vi "2 Sync - Digital Trigger.vi"() -> ()   [LabVIEW 2023]
doc: "This example demonstrates how to acquire a single buffer of voltage measurements using a DAQmx device.\n\nFor instructions on how to connect your signals to the DAQ device, refer to your device documentation."
uses:
  <vilib>/DAQmx/create/channels.llb/DAQmx Create Channel (AI-Voltage-Basic).vi
  <vilib>/DAQmx/configure/timing.llb/DAQmx Timing (Sample Clock).vi
  <vilib>/DAQmx/read.llb/DAQmx Read (Analog Wfm 1Chan NSamp).vi
  <vilib>/Analysis/NI_AALBase.lvlib
  <resource>/objmgr/daqmx.rc
  <vilib>/DAQmx/configure/trigger.llb/DAQmx Start Trigger (Digital Edge).vi
  <vilib>/DAQmx/write.llb/DAQmx Write (Digital Bool 1Line 1Point).vi
  <vilib>/DAQmx/configure/timing.llb/DAQmx Timing (Implicit).vi
  <vilib>/DAQmx/create/channels.llb/DAQmx Create Channel (CO-Pulse Generation-Frequency).vi
  <vilib>/DAQmx/create/channels.llb/DAQmx Create Channel (DO-Digital Output).vi
panel:
  in  "Trigger Output: Line":tag="MIODAQ/port0/line2"
  in  "Device 2: Trigger Input":tag="/cDAQ9189-2628AACMod5/PFI4"
  in  "Device 1: Trigger Input":tag="/MIODAQ/PFI4"
  in  "Square Wave Output: Terminal":tag="/MIODAQ/PFI0"
  in  "Square Wave Output: Source":tag="MIODAQ/ctr0"
  out "Progress":i32(slide) scale=0.0..9.0
  out "Standard Deviation":dbl format="%0.2f"
  out "Range":dbl
  out "Mean":dbl format="%0.2f"
  out "Skew":dbl
  in  "Device 2: Analog Input Channel":tag="cDAQ9189-2628AACMod1/ai0"
  out "Waveform Graph":waveform(dbl)[](graph)
  in  "Device 1: Analog Input Channel":tag="MIODAQ/ai0"
  # "Channel Settings"
  # "Acquired Data"
  # "Trigger Acq Settings"
  # "Output Signal Settings"
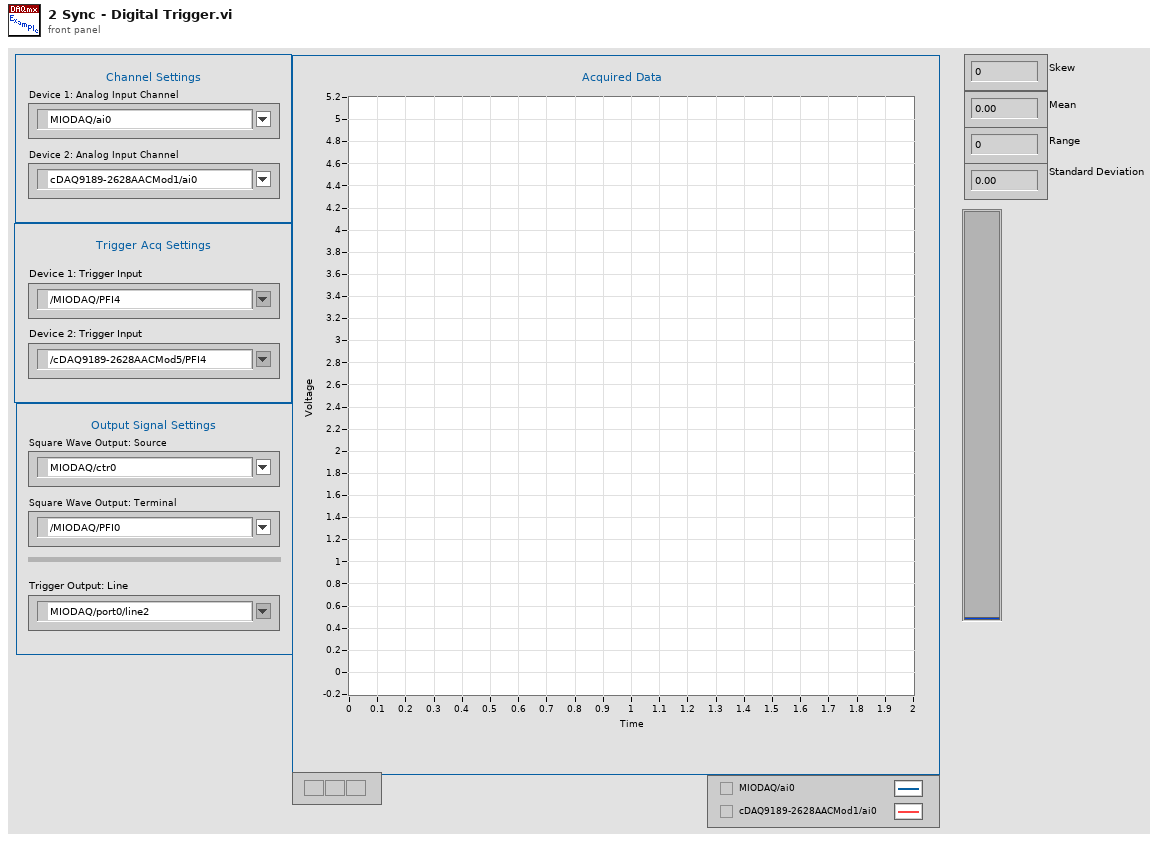
[diagram p1: front panel]
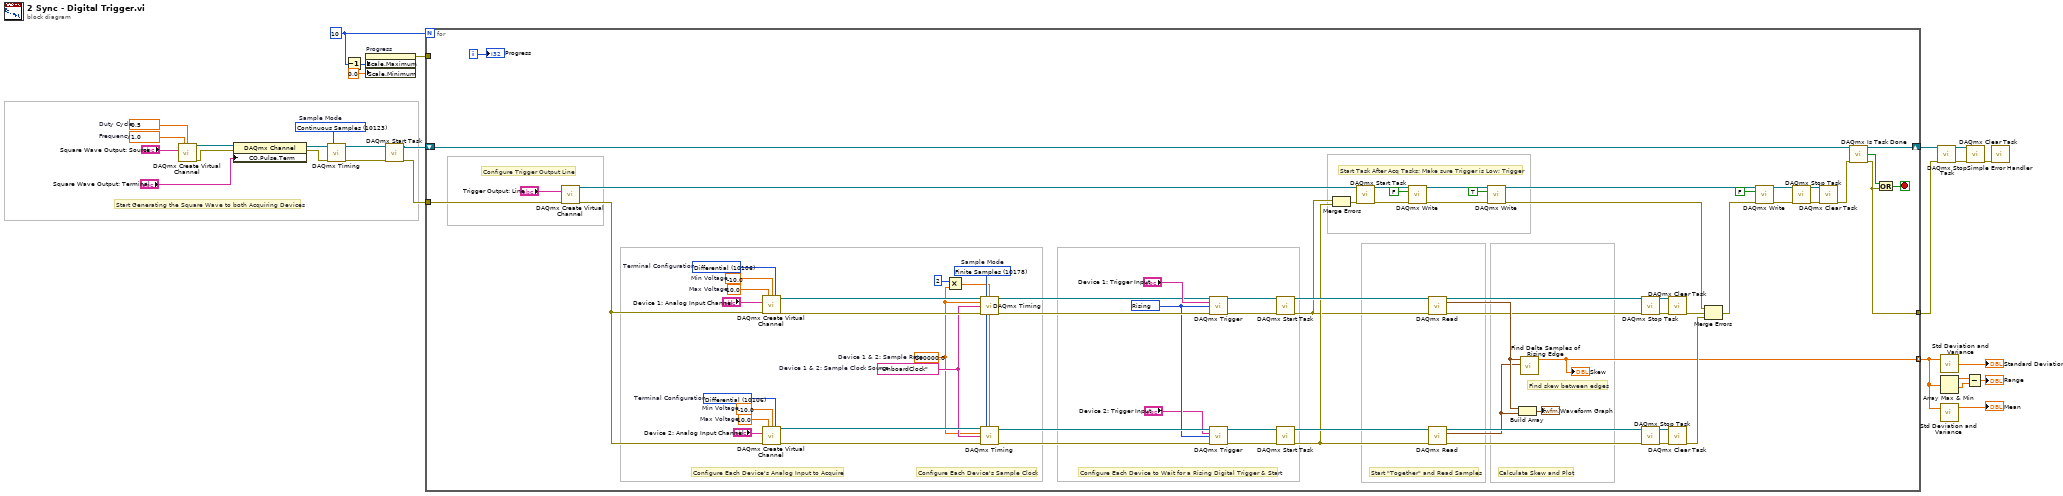
[diagram p0: block diagram]
diagram:
  w16 = 1.0  # Frequency
  w17 = 0.5  # Duty Cycle
  w9 = 10123 items=["Finite Samples"=10178, "Continuous Samples"=10123, "Hardware Timed Single Point"=12522]  # Sample Mode
  w22 = 10
  # "Start Generating the Square Wave to both Acquiring Devices"
  n1 = call-poly <vilib>:"DAQmx Create Virtual Channel.vi"("frequency"=w16, "duty cycle"=w17, "counter"="Square Wave Output: Source") -> ("task out"=w11:refnum<k21>, "error out"=w12:errorcluster)  [unwired: 11 in]
  n2 = property class="DAQmx Channel"(reference=w11, error in=w12, "CO.Pulse.Term"="Square Wave Output: Terminal") -> (reference out=w15:refnum<k21>, error out=w14:errorcluster)
  n3 = call-poly <vilib>:"DAQmx Timing.vi"("task/channels in"=w15, "sample mode"=w9, "error in"=w14) -> ("task out"=w19:refnum<k21>, "error out"=w18:errorcluster)  [unwired: 11 in]
  n4 = Decrement(x=w22) -> (x-1=w2:i32)
  n5 = property on="Progress" class="Slide (strict)"("Scale.Maximum"=w2, "Scale.Minimum"=0.0 ("Scale.Range:Minimum")) -> (error out=w20:errorcluster)  [unwired: 2 in, 1 out]
  n6 = call <vilib>:"DAQmx Start Task.vi"("task/channels in"=w19, "error in"=w18) -> ("task out"=w6:refnum<k21>, "error out"=w1:errorcluster)  [unwired: 12 in]
  n7 = for {
    N: w22 -> [_]
    tunnel: [w62] -> w24 mode=indexing
    tunnel: w20 -> [_]
    tunnel: [w70] -> w4
    shift-right: [w67] -> w5
    shift-left: w6 -> [w66]
    tunnel: w1 -> [w51]
    i -> [w75]
    stop <- w68 stop-if-true
    w65 = 100000.0  # Device 1 & 2: Sample Rate
    w84 = tag "OnboardClock"  # Device 1 & 2: Sample Clock Source
    w54 = 10280 items=["Rising"=10280, "Falling"=10171] ("Digital Start Trigger Edge")
    w90 = 10.0  # Max Voltage
    w89 = -10.0  # Min Voltage
    w88 = 10106 items=["default"=-1, "RSE"=10083, "NRSE"=10078, "Differential"=10106, "Pseudodifferential"=12529]  # Terminal Configuration
    w94 = 10.0  # Max Voltage
    w95 = -10.0  # Min Voltage
    w96 = 10106 items=["default"=-1, "RSE"=10083, "NRSE"=10078, "Differential"=10106, "Pseudodifferential"=12529]  # Terminal Configuration
    w74 = 10178 items=["Finite Samples"=10178, "Continuous Samples"=10123, "Hardware Timed Single Point"=12522]  # Sample Mode
    # "Start Task After Acq Tasks; Make sure Trigger is Low; Trigger"
    # "Configure Each Device to Wait for a Rising Digital Trigger & Start"
    # "Configure Trigger Output Line"
    # "Calculate Skew and Plot"
    # "Start \"Together\" and Read Samples"
    # "Configure Each Device's Sample Clock"
    # "Configure Each Device's Analog Input to Acquire"
    # "Find skew between edges"
    n8 = call-poly <vilib>:"DAQmx Create Virtual Channel.vi"("lines"="Trigger Output: Line", "error in"=w51) -> ("task out"=w43:refnum<k21>, "error out"=w50:errorcluster)  [unwired: 12 in]
    n9 = call-poly <vilib>:"DAQmx Create Virtual Channel.vi"("maximum value"=w94, "minimum value"=w95, "input terminal configuration"=w96, "physical channels"="Device 1: Analog Input Channel", "error in"=w50) -> ("task out"=w99:refnum<k21>, "error out"=w100:errorcluster)  [unwired: 9 in]
    n10 = call-poly <vilib>:"DAQmx Create Virtual Channel.vi"("maximum value"=w90, "minimum value"=w89, "input terminal configuration"=w88, "physical channels"="Device 2: Analog Input Channel", "error in"=w50) -> ("task out"=w87:refnum<k21>, "error out"=w86:errorcluster)  [unwired: 9 in]
    n11 = Multiply(x=2, y=w65) -> (x*y=w63:dbl)
    n12 = call-poly <vilib>:"DAQmx Timing.vi"("task/channels in"=w99, "sample mode"=w74, "samples per channel"=w63, "rate"=w65, "source"=w84, "error in"=w100) -> ("task out"=w60:refnum<k21>, "error out"=w59:errorcluster)  [unwired: 8 in]
    n13 = call-poly <vilib>:"DAQmx Timing.vi"("task/channels in"=w87, "sample mode"=w74, "samples per channel"=w63, "rate"=w65, "source"=w84, "error in"=w86) -> ("task out"=w57:refnum<k21>, "error out"=w55:errorcluster)  [unwired: 8 in]
    n14 = call-poly <vilib>:"DAQmx Trigger.vi"("task/channels in"=w60, "source"="Device 1: Trigger Input", "edge"=w54, "error in"=w59) -> ("task out"=w58:refnum<k21>, "error out"=w41:errorcluster)  [unwired: 10 in]
    n15 = call-poly <vilib>:"DAQmx Trigger.vi"("task/channels in"=w57, "source"="Device 2: Trigger Input", "edge"=w54, "error in"=w55) -> ("task out"=w56:refnum<k21>, "error out"=w42:errorcluster)  [unwired: 10 in]
    n16 = call <vilib>:"DAQmx Start Task.vi"("task/channels in"=w58, "error in"=w41) -> ("task out"=w98:refnum<k21>, "error out"=w39:errorcluster)  [unwired: 12 in]
    n17 = call <vilib>:"DAQmx Start Task.vi"("task/channels in"=w56, "error in"=w42) -> ("task out"=w79:refnum<k21>, "error out"=w40:errorcluster)  [unwired: 12 in]
    n18 = Merge Errors(w39, w40) -> (w38:errorcluster)
    n19 = call <vilib>:"DAQmx Start Task.vi"("task/channels in"=w43, "error in"=w38) -> ("task out"=w49:refnum<k21>, "error out"=w48:errorcluster)  [unwired: 12 in]
    n20 = call-poly <vilib>:"DAQmx Write.vi"("task/channels in"=w49, "data"=FALSE, "error in"=w48) -> ("task out"=w45:refnum<k21>, "error out"=w44:errorcluster)  [unwired: 10 in, 1 out]
    n21 = call-poly <vilib>:"DAQmx Read.vi"("task/channels in"=w98, "error in"=w39) -> ("task out"=w91:refnum<k21>, "data"=w77:waveform(dbl), "error out"=w71:errorcluster)  [unwired: 11 in]
    n22 = call-poly <vilib>:"DAQmx Read.vi"("task/channels in"=w79, "error in"=w40) -> ("task out"=w82:refnum<k21>, "data"=w76:waveform(dbl), "error out"=w83:errorcluster)  [unwired: 11 in]
    n23 = call-poly <vilib>:"DAQmx Write.vi"("task/channels in"=w45, "data"=TRUE, "error in"=w44) -> ("task out"=w31:refnum<k21>, "error out"=w37:errorcluster)  [unwired: 10 in, 1 out]
    n24 = Build Array(w77, w76) -> (→"Waveform Graph":waveform(dbl)[])
    n25 = call "Find Delta Samples of Rising Edge.vi"("Channel 2"=w76, "Channel 1"=w77) -> ("Sample Offset"=w62:dbl)  [unwired: 9 in]
    "Skew" <- w62
    n26 = call <vilib>:"DAQmx Stop Task.vi"("task/channels in"=w91, "error in"=w71) -> ("task out"=w93:refnum<k21>, "error out"=w92:errorcluster)  [unwired: 12 in]
    n27 = call <vilib>:"DAQmx Stop Task.vi"("task/channels in"=w82, "error in"=w83) -> ("task out"=w80:refnum<k21>, "error out"=w81:errorcluster)  [unwired: 12 in]
    n28 = call <vilib>:"DAQmx Clear Task.vi"("task in"=w93, "error in"=w92) -> ("error out"=w72:errorcluster)  [unwired: 13 in]
    n29 = call <vilib>:"DAQmx Clear Task.vi"("task in"=w80, "error in"=w81) -> ("error out"=w73:errorcluster)  [unwired: 13 in]
    n30 = Merge Errors(w37, w72, w73) -> (w30:errorcluster)
    n31 = call-poly <vilib>:"DAQmx Write.vi"("task/channels in"=w31, "data"=FALSE, "error in"=w30) -> ("task out"=w32:refnum<k21>, "error out"=w33:errorcluster)  [unwired: 10 in, 1 out]
    n32 = call <vilib>:"DAQmx Stop Task.vi"("task/channels in"=w32, "error in"=w33) -> ("task out"=w36:refnum<k21>, "error out"=w35:errorcluster)  [unwired: 12 in]
    n33 = call <vilib>:"DAQmx Clear Task.vi"("task in"=w36, "error in"=w35) -> ("error out"=w29:errorcluster)  [unwired: 13 in]
    n34 = call <vilib>:"DAQmx Is Task Done.vi"("task/channels in"=w66, "error in"=w29) -> ("task out"=w67:refnum<k21>, "task done?"=w69:bool, "error out"=w70:errorcluster)  [unwired: 11 in]
    n35 = Compound Arithmetic op=OR(w69, w70) -> (w68:bool)
    "Progress" <- w75
  }
  n36 = call <vilib>:"DAQmx Stop Task.vi"("task/channels in"=w5, "error in"=w4) -> ("task out"=w7:refnum<k21>, "error out"=w8:errorcluster)  [unwired: 12 in]
  n37 = call <vilib>:"Std Deviation and Variance.vi"("X"=w24) -> ("standard deviation"=→"Standard Deviation":dbl)  [unwired: 1 in, 2 out]
  n38 = Array Max & Min(array=w24) -> (max value=w28:dbl, min value=w27:dbl)  [unwired: 2 out]
  n39 = call <vilib>:"Std Deviation and Variance.vi"("X"=w24) -> ("mean"=→"Mean":dbl)  [unwired: 1 in, 2 out]
  n40 = Subtract(x=w28, y=w27) -> (x-y=→"Range":dbl)
  n41 = call <vilib>:"DAQmx Clear Task.vi"("task in"=w7, "error in"=w8) -> ("error out"=w3:errorcluster)  [unwired: 13 in]
  n42 = call <vilib>:"Simple Error Handler.vi"("error in (no error)"=w3) -> ()  [unwired: 4 in, 5 out]
